vi "transition.vi"(8 "error in (no error)":errorcluster, 10 "ContextData In":refnum<class "ContextData.lvclass">, 11 "Run in":refnum<class "Initialize References.lvclass">) -> (0 "error out":errorcluster, 2 "ContextData Out":refnum<class "ContextData.lvclass">, 3 "Next Step":refnum<class "State.lvclass">)   [LabVIEW 2019, in "Initialize References.lvclass"]
uses:
  Initialize References.lvclass
  State/State.lvclass
  ContextData/ContextData.lvclass
  Launch UI/Launch UI.lvclass
  C:/Users/fflores/Documents/GitHub Projects/Simon/Simon Game/OOP States/State/State.lvclass
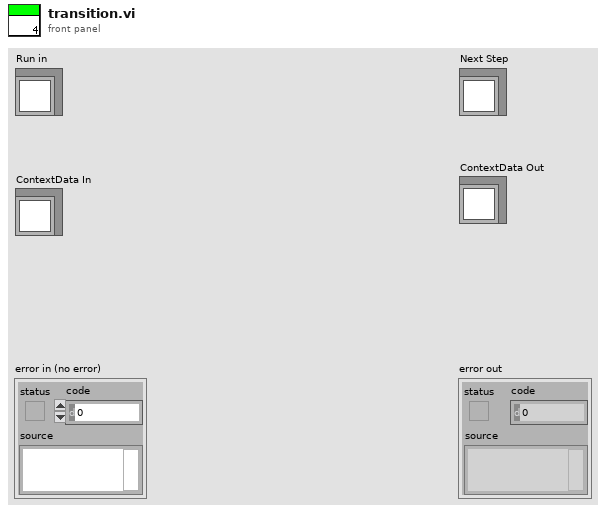
[diagram p1: front panel]
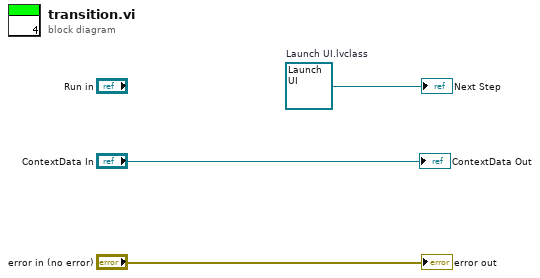
[diagram p0: block diagram]
diagram:
  w1 = refnum<class "Launch UI.lvclass"> refnum  # Launch UI.lvclass
  "error out" <- "error in (no error)"
  "Next Step" <- w1
  "ContextData Out" <- "ContextData In"
